vi "PG_factor.vi"(8 "error in (no error)":errorcluster, 11 "SI656 in":refnum<class "SI656.lvclass">) -> (0 "error out":errorcluster, 2 "PG Factor":dbl, 3 "SI656 out":refnum<class "SI656.lvclass">)   [LabVIEW 2022 SP3, in "SI656.lvclass"]
uses:
  SI656.lvclass
  SI656.lvclass/SI656.ctl
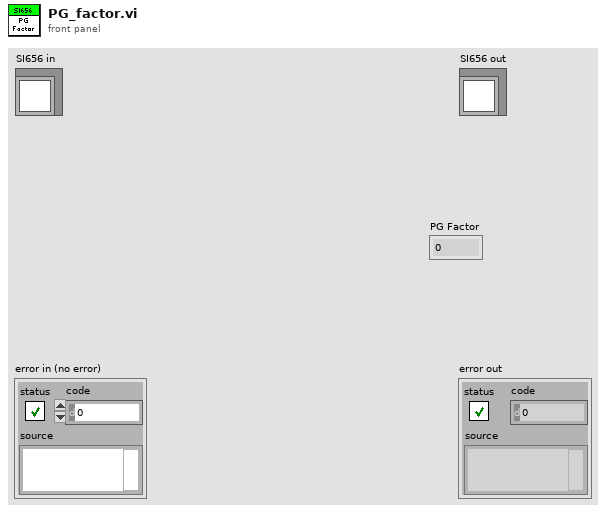
[diagram p1: front panel]
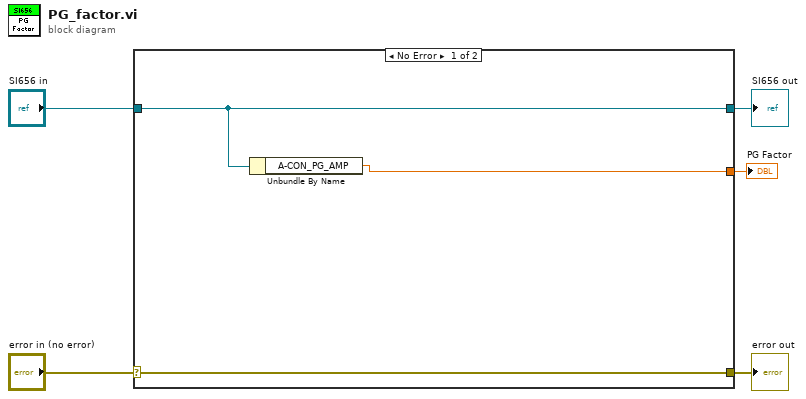
[diagram p0: block diagram]
diagram:
  n1 = case shown="No Error" "error in (no error)" {
    selector: "error in (no error)" -> [w8 w10]
    tunnel: [w8 w10] -> w4
    tunnel: [w7 w9] -> w2
    tunnel: "SI656 in" -> [w7 w9]
    tunnel: [w6 _] -> w1
    frame No Error {
      n2 = Unbundle By Name(w7) -> ("A-CON_PG_AMP"=w6:dbl)
    }
    frame Error {
    }
  }
  "error out" <- w4
  "SI656 out" <- w2
  "PG Factor" <- w1
